vi "labview_test.vi"() -> ()   [LabVIEW 2021]
uses:
  <vilib>/Utility/file.llb/Read Delimited Spreadsheet (DBL).vi
  <vilib>/Analysis/Matrix/Numeric/Conversions/Array To Matrix - RA2.vi
  <vilib>/Analysis/Matrix/Numeric/Conversions/Matrix To Array - CM.vi
  <vilib>/Analysis/Matrix/NI_Matrix.lvlib
panel:
  out "mae values":cdb
  out "mae Vectors":cdb
  out "Difference Eigenvectors":cdb[][](array[numeric])
  out "Difference Eigenvalues":cdb[](array[numeric])
  out "LabVIEWEigenvectors":cdb[][](array[numeric])
  out "LabveiwEigenvalues":cdb[](array[numeric])
  out "Elapsed time":dbl=0.5790897820043028
  out "ScipyEigenvectors":dbl[][](array[numeric])
  out "ScipyEigenvalues":dbl[](array[numeric])
  out "standard output":string
  out "standard error":string
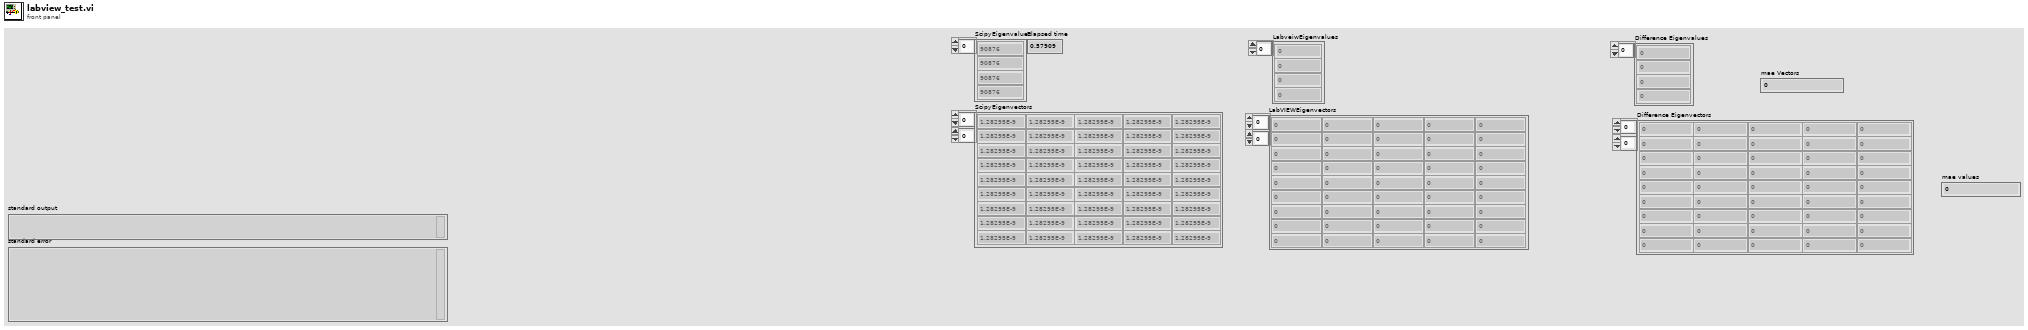
[diagram p1: front panel]
types:
  T1 = typedef "NI_Matrix.lvlib/RealMatrix.ctl" = dbl[][]
  T2 = typedef "NI_Matrix.lvlib/ComplexMatrix.ctl" = cdb[][]
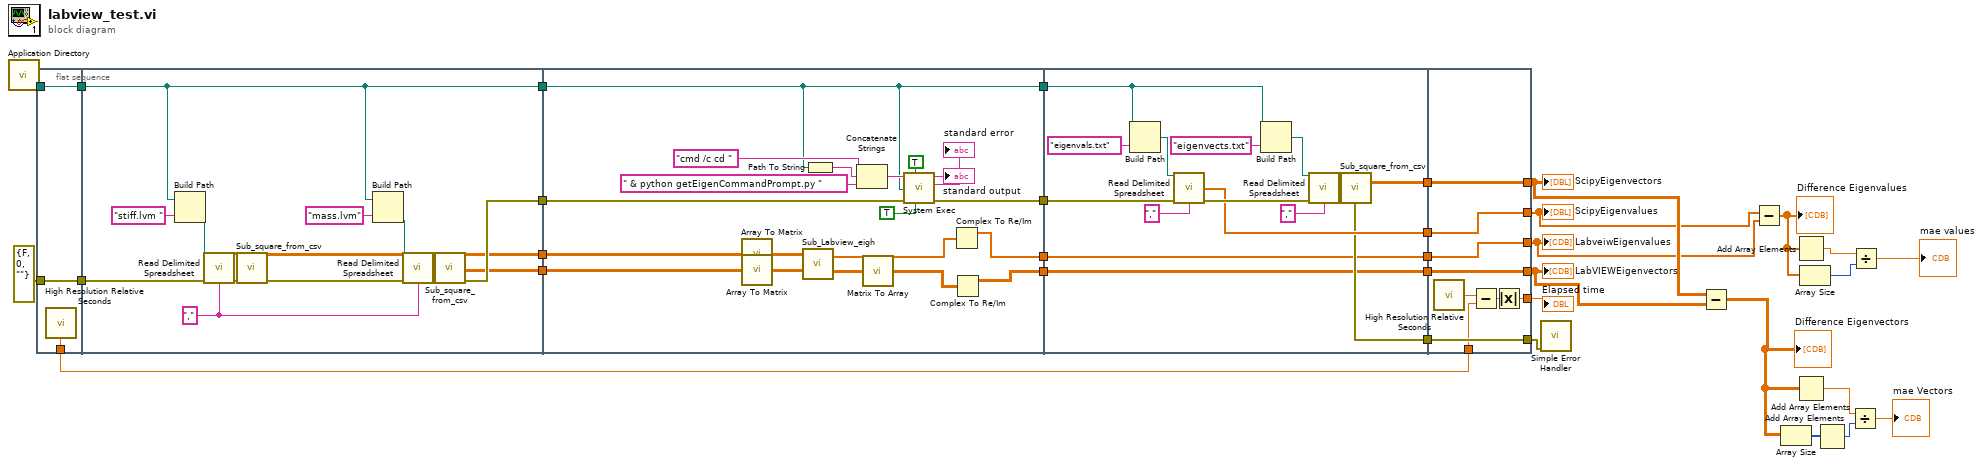
[diagram p0: block diagram]
diagram:
  n1 = call <vilib>:"Application Directory.vi"() -> ("Application Directory"=w31:path)
  n2 = flat-sequence {
    tunnel: errorcluster {"status"=FALSE, "code"=0, "source"=""} ("error in (no error)") -> [w35]
    tunnel: w31 -> [w36]
    tunnel: [w36] -> w27
    tunnel: [w35] -> w28
    tunnel: [w34] -> w15
    tunnel: w28 -> [w42]
    tunnel: w27 -> [w47]
    tunnel: [w47] -> w24
    tunnel: [w41] -> w23
    tunnel: [w39] -> w22
    tunnel: [w37] -> w21
    tunnel: [w67] -> w33
    tunnel: w24 -> [w61]
    tunnel: [w61] -> w32
    tunnel: w23 -> [w68]
    tunnel: w22 -> [w58]
    tunnel: [w50] -> w26
    tunnel: [w51] -> w25
    tunnel: w21 -> [w54]
    tunnel: w33 -> [w84]
    tunnel: w32 -> [w82]
    tunnel: [w77] -> w20
    tunnel: [w74] -> w19
    tunnel: w26 -> [w73]
    tunnel: w25 -> [w72]
    tunnel: [w73] -> w18
    tunnel: [w72] -> w17
    tunnel: [w70] -> w16
    tunnel: w16 -> [w93]
    tunnel: w20 -> [w92]
    tunnel: w19 -> [w91]
    tunnel: [w93] -> w13
    tunnel: [w92] -> w11
    tunnel: [w91] -> w29
    tunnel: [w90] -> w12
    tunnel: w17 -> [w90]
    tunnel: w18 -> [w89]
    tunnel: [w89] -> w10
    tunnel: w15 -> [w88]
    tunnel: [w85] -> w14
    frame #0 {
      n3 = call <vilib>:"High Resolution Relative Seconds.vi"() -> ("relative seconds"=w34:dbl)
    }
    frame #1 {
      w44 = "," ("delimiter (\\t)")
      n4 = Build Path(base path=w47, name or relative path="stiff.lvm ") -> (appended path=w46:path)
      n5 = call-poly <vilib>:"Read Delimited Spreadsheet.vi"("file path (dialog if empty)"=w46, "error in (no error)"=w42, "delimiter (\\t)"=w44) -> ("all rows"=w40:dbl[][], "error out"=w43:errorcluster)  [unwired: 7 in, 4 out]
      n6 = call "Sub_square_from_csv.vi"("To Flattened"=w40) -> ("Square"=w37:dbl[][])  [unwired: 10 in]
      n7 = Build Path(base path=w47, name or relative path="mass.lvm") -> (appended path=w45:path)
      n8 = call-poly <vilib>:"Read Delimited Spreadsheet.vi"("file path (dialog if empty)"=w45, "error in (no error)"=w43, "delimiter (\\t)"=w44) -> ("all rows"=w38:dbl[][], "error out"=w41:errorcluster)  [unwired: 7 in, 4 out]
      n9 = call "Sub_square_from_csv.vi"("To Flattened"=w38) -> ("Square"=w39:dbl[][])  [unwired: 10 in]
    }
    frame #2 {
      n10 = call-poly <vilib>:"Array To Matrix.vi"("Real 2D Array"=w54) -> ("Real Matrix"=w56:T1)
      n11 = call-poly <vilib>:"Array To Matrix.vi"("Real 2D Array"=w58) -> ("Real Matrix"=w57:T1)
      n12 = call "Sub_Labview_eigh.vi"("Mass"=w57, "Stiffness"=w56) -> ("Eigenvectors"=w55:T2, "Eigenvalues"=w53:cdb[])
      n13 = Path To String(path=w61) -> (string=w60:string)
      n14 = Concatenate Strings("cmd /c cd " ("command line"), w60, " & python getEigenCommandPrompt.py " ("standard input")) -> (w62:string)
      n15 = call-poly <vilib>:"Matrix To Array.vi"("Complex Matrix"=w55) -> ("Complex 2D Array"=w52:cdb[][])
      n16 = call <vilib>:"System Exec.vi"("run minimized? (F)"=TRUE, "wait until completion? (T)"=TRUE, "error in (no error)"=w68, "working directory"=w61, "command line"=w62) -> ("error out"=w67:errorcluster, "standard error"=→"standard error":string, "standard output"=→"standard output":string)  [unwired: 3 in, 1 out]
      n17 = Complex To Re/Im(x + iy=w53) -> (x=w50:dbl[])  [unwired: 1 out]
      n18 = Complex To Re/Im(x + iy=w52) -> (x=w51:dbl[][])  [unwired: 1 out]
    }
    frame #3 {
      n19 = Build Path(base path=w82, name or relative path="eigenvals.txt") -> (appended path=w81:path)
      n20 = call-poly <vilib>:"Read Delimited Spreadsheet.vi"("file path (dialog if empty)"=w81, "error in (no error)"=w84, "delimiter (\\t)"="," ("delimiter (\\t)")) -> ("first row"=w77:dbl[], "error out"=w83:errorcluster)  [unwired: 7 in, 4 out]
      n21 = Build Path(base path=w82, name or relative path="eigenvects.txt") -> (appended path=w80:path)
      n22 = call-poly <vilib>:"Read Delimited Spreadsheet.vi"("file path (dialog if empty)"=w80, "error in (no error)"=w83, "delimiter (\\t)"="," ("delimiter (\\t)")) -> ("all rows"=w71:dbl[][], "error out"=w74:errorcluster)  [unwired: 7 in, 4 out]
      n23 = call "Sub_square_from_csv.vi"("To Flattened"=w71) -> ("Square"=w70:dbl[][])  [unwired: 10 in]
    }
    frame #4 {
      n24 = call <vilib>:"High Resolution Relative Seconds.vi"() -> ("relative seconds"=w87:dbl)
      n25 = Subtract(x=w87, y=w88) -> (x-y=w86:dbl)
      n26 = Absolute Value(x=w86) -> (abs(x)=w85:dbl)
    }
  }
  n27 = call <vilib>:"Simple Error Handler.vi"("error in (no error)"=w29) -> ()  [unwired: 4 in, 5 out]
  n28 = Subtract(x=w13, y=w12) -> (x-y=w9:dbl[][])
  "Difference Eigenvectors" <- w9
  n29 = Subtract(x=w11, y=w10) -> (x-y=w8:dbl[])
  "Difference Eigenvalues" <- w8
  n30 = Array Size(array=w9) -> (size(s)=w4:i32[])
  n31 = Add Array Elements(numeric array=w8) -> (sum=w6:dbl)
  n32 = Add Array Elements(numeric array=w9) -> (sum=w5:dbl)
  n33 = Array Size(array=w8) -> (size(s)=w7:i32)
  n34 = Add Array Elements(numeric array=w4) -> (sum=w3:i32)
  n35 = Divide(x=w5, y=w3) -> (x/y=→"mae Vectors":dbl)
  n36 = Divide(x=w6, y=w7) -> (x/y=→"mae values":dbl)
  "ScipyEigenvalues" <- w11
  "ScipyEigenvectors" <- w13
  "Elapsed time" <- w14
  "LabveiwEigenvalues" <- w10
  "LabVIEWEigenvectors" <- w12
